vi "slscsl_relayControl.vi"(8 "error in (no error)":errorcluster, 9 "RelayAction":T1=21 items=["CloseRelay"=21, "OpenRelay"=20], 10 "relayNames":string, 11 "slscsl in":refnum<class "slscsl.lvclass">) -> (0 "error out":errorcluster, 2 "switchActionArray":T2 {"RelayAction" items=["CloseRelay"=21, "OpenRelay"=20]}, 3 "slscsl out":refnum<class "slscsl.lvclass">)   [LabVIEW 2016, in "SLSC Switch.lvlib" / "slscsl.lvclass"]
uses:
  slscsl.lvclass
  SwitchActionsArray.ctl
  SwitchAction.ctl
  RelayAction.ctl
  slscsl.lvclass/slscsl.ctl
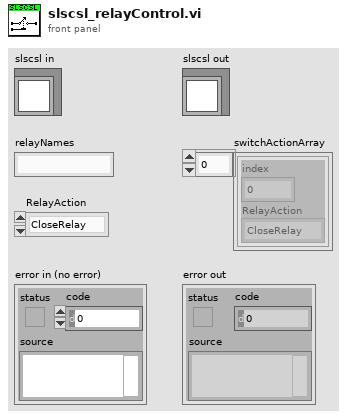
[diagram p1: front panel]
types:
  T1 = typedef "SLSC Switch.lvlib/slscsl.lvclass/RelayAction.ctl" = u32
  T2 = typedef "SLSC Switch.lvlib/slscsl.lvclass/SwitchActionsArray.ctl" = T3[]
  T3 = typedef "SLSC Switch.lvlib/slscsl.lvclass/SwitchAction.ctl" = cluster{"index":i32, "RelayAction":T1}
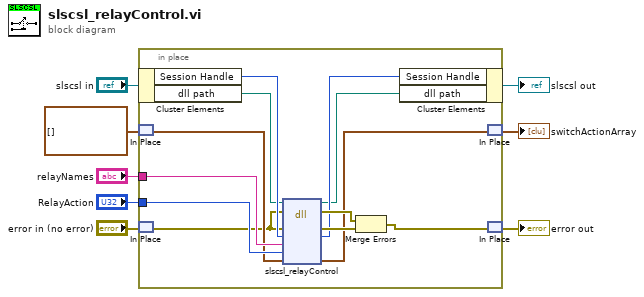
[diagram p0: block diagram]
diagram:
  n1 = in-place {
    in-place-border: "relayNames" -> [w16]
    in-place-border: "RelayAction" -> [w15]
    n2 = in-place-cluster #1("slscsl in") -> ("Session Handle"=w18:u64, "dll path"=w10:path)
    n3 = in-place-match #2(T2 [] ("SwitchActionList")) -> (w14:T2)
    n4 = in-place-match #3("error in (no error)") -> (w12:errorcluster)
    n5 = dll-call lib="?" fn="slscsl_relayControl"(path in=w10, error in=w12, "errorCluster"=w12, "sessionHandle"=w18, "relayNames"=w16, "relayActions"=w15, "switchActionArray"=w14) -> (path out=w9:path, error out=w20:errorcluster, "errorCluster"=w19:errorcluster, "sessionHandle"=w17:u64, "switchActionArray"=w13:T2)  [unwired: 4 in]
    n6 = Merge Errors(w20, w19) -> (w11:errorcluster)
    n7 = in-place-cluster #1("Session Handle"=w17, "dll path"=w9) -> (→"slscsl out":refnum<class "slscsl.lvclass">)
    n8 = in-place-match #2(w13) -> (→"switchActionArray":T2)
    n9 = in-place-match #3(w11) -> (→"error out":errorcluster)
  }
